vi "TildaPassiveTrigger.vi"() -> (15 "beamGateFallingEdge":bool, 18 "triggered":bool)   [LabVIEW 2014]
uses:
  Controls/triggerEdge.ctl
  <vilib>/rvi/eio/common/nirviEmuTemplateMethod_errors.vi
  Trigger/triggerGlobalVars.vi
  <vilib>/eio/EIONode/EIONode.xnode
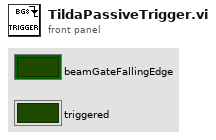
[diagram p1: front panel]
types:
  T1 = typedef "triggerEdge.ctl" = enum8{"either", "false-true", "true-false"}
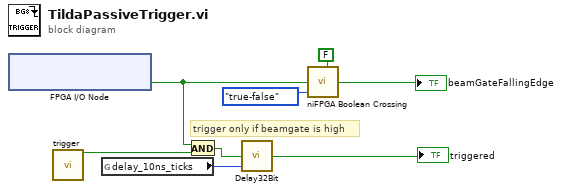
[diagram p0: block diagram]
diagram:
  # "trigger only if beamgate is high"
  n1 = xnode "FPGA I/O Node"() -> ("Connector1/DIO25"=w5:bool)  [unwired: 1 in, 1 out]
  n2 = call "trigger.vi"() -> ("triggered"=w8:bool)  [unwired: 19 in]
  n3 = global read "triggerGlobalVars.vi" "delay_10ns_ticks"() -> (w6:u32)
  n4 = And(x=w5, y=w8) -> (x .and. y?=w7:bool)
  n5 = call "Delay32Bit.vi"("delay(ticks)"=w6, "In"=w7) -> ("Out"=→"triggered":bool)  [unwired: 3 in]
  n6 = call <vilib>:"niFPGA Boolean Crossing.vi"("input"=w5, "triggerEdge"=triggerEdge."true-false", "initialize"=FALSE) -> ("crossing"=→"beamGateFallingEdge":bool)  [unwired: 6 in]
